vi "Configure Channels.vi"(8 "error in":errorcluster, 11 "DIO DAQmx PWM CFG in":refnum<class "CO DAQmx PWM CFG.lvclass">) -> (0 "error out":errorcluster, 3 "DIO DAQmx PWM CFG out":refnum<class "CO DAQmx PWM CFG.lvclass">)   [LabVIEW 2023, in "CO DAQmx PWM CFG.lvclass"]
uses:
  CO DAQmx PWM CFG.lvclass
  CO DAQmx PWM CFG.lvclass/CO DAQmx PWM CFG.ctl
  <vilib>/Utility/error.llb/Error Cluster From Error Code.vi
  <vilib>/ErrorRing/Error Ring.xnode
  Configuration/Configuration JSON/Configuration JSON Base/CFG JSON.lvclass
  DAQmx/DAQmx Base CFG/DAQmx Base CFG.lvclass
  <vilib>/DAQmx/create/channels.llb/DAQmx Create Channel (CO-Pulse Generation-Frequency).vi
  9b4e2dbf-c434-4eef-b69c-50b2f8d92478.vi
panel:
  out "Idle State":i32(ring)=10214 items=["High"=10192, "Low"=10214]
  out "Units":i32(ring)=10373 items=["Hz"=10373]
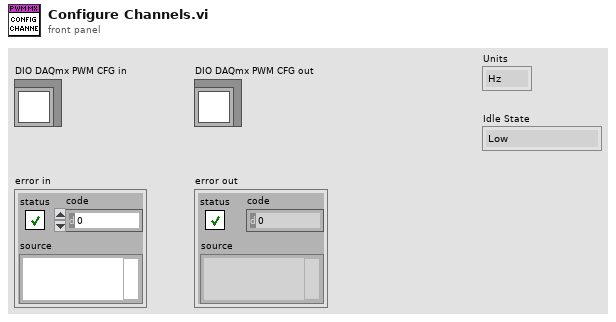
[diagram p1: front panel]
types:
  T1 = cluster{"Name":string, "Enabled":bool, "Duty Cycle":dbl, "Frequency":dbl, "Units":string, "Idle State":string, "Initial Delay":dbl}[]
  T2 = typedef "LVStringsAndValuesArrayTypeDef_I32.ctl" = cluster{"String":string, "Value":i32}[]
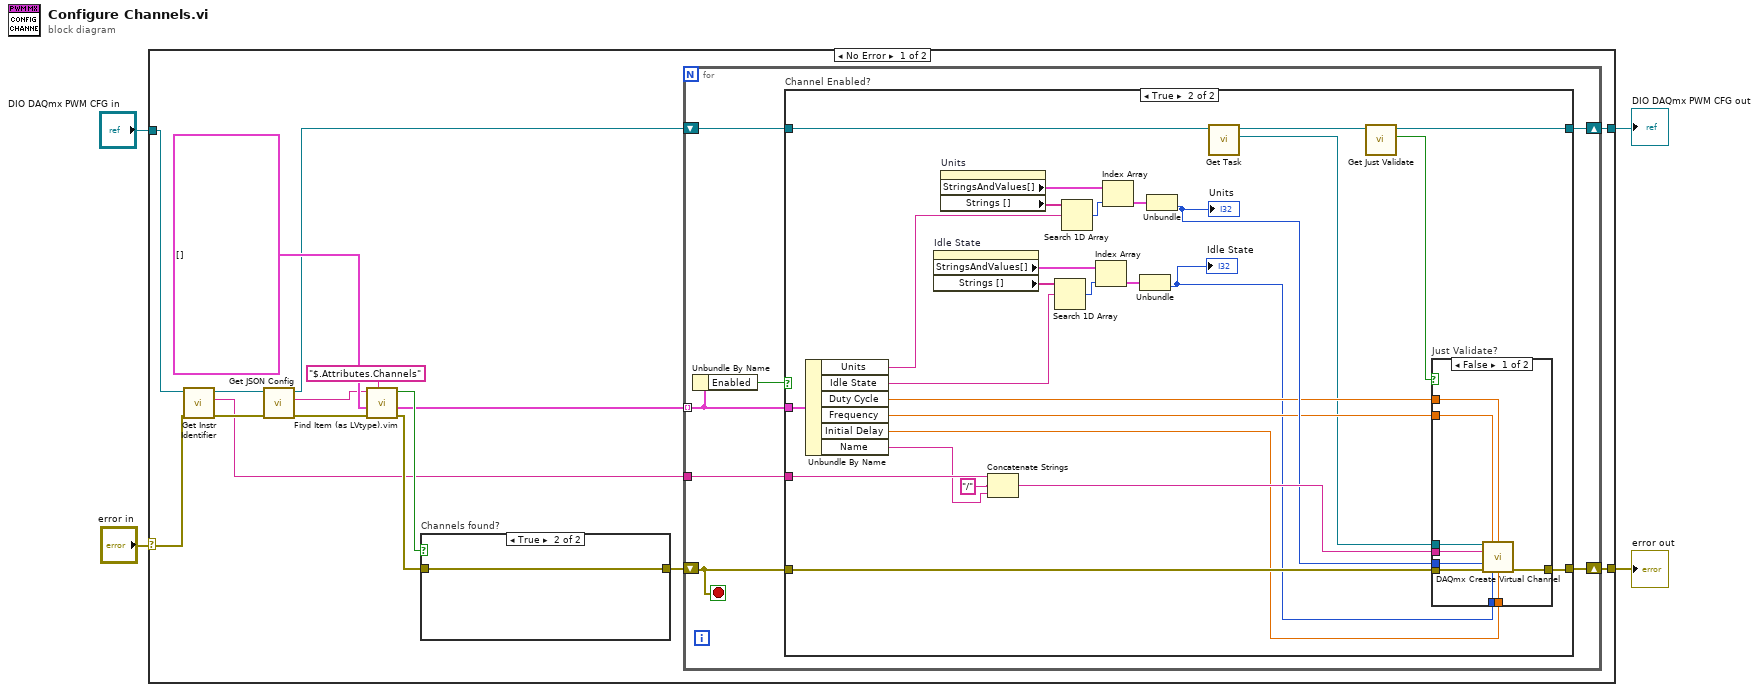
[diagram p0: block diagram]
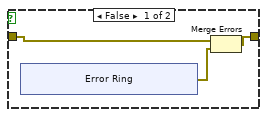
[diagram p4: hidden frame]
diagram:
  n1 = case shown="No Error" "error in" {
    selector: "error in" -> [w5 w76]
    tunnel: "DIO DAQmx PWM CFG in" -> [w9 w77]
    tunnel: [w8 w76] -> w3
    tunnel: [w6 w77] -> w2
    frame No Error {
      n2 = call-dynamic "Get Instr Identifier.vi"("error in (no error)"=w5, "Configuration Base in"=w9) -> ("error out"=w12:errorcluster, "Instr Ident"=w10:string, "Configuration Base out"=w11:refnum<class "CO DAQmx PWM CFG.lvclass">)  [unwired: 7 in]
      n3 = call "Get JSON Config.vi"("error in (no error)"=w12, "CFG Base in"=w11) -> ("error out"=w19:errorcluster, "<JSON>Config>"=w13:string, "CFG Base out"=w7:refnum<class "CO DAQmx PWM CFG.lvclass">)  [unwired: 7 in]
      n4 = call "Find Item (as LVtype).vim"("$Path or Item Name"="$.Attributes.Channels", "error in (no error)"=w19, "Data Type and Default Value"=T1 [], "JSON"=w13) -> ("error out"=w17:errorcluster, "Data"=w15:T1, "Found"=w18:bool)  [unwired: 4 in, 1 out]
      n5 = case "Channels found?" shown="True" w18 {
        tunnel: w17 -> [w69 w75]
        tunnel: [w67 w75] -> w16
        frame False {
          n6 = xnode "Error Ring"() -> ("error out"=w68:errorcluster)
          n7 = Merge Errors(w69, w68) -> (w67:errorcluster)
        }
        frame True {
        }
      }
      n8 = for {
        tunnel: w15 -> [w24] mode=indexing
        shift-right: [w27] -> w8
        shift-left: w16 -> [w26]
        tunnel: w10 -> [w25]
        shift-right: [w22] -> w6
        shift-left: w7 -> [w21]
        stop <- w26 stop-if-true
        n9 = Unbundle By Name(w24) -> ("Enabled"=w23:bool)
        n10 = case "Channel Enabled?" shown="True" w23 {
          tunnel: [w29 w34] -> w27
          tunnel: w26 -> [w29 w49]
          tunnel: w25 -> [_ w47]
          tunnel: w24 -> [_ w45]
          tunnel: [w28 w31] -> w22
          tunnel: w21 -> [w28 w32]
          frame False {
          }
          frame True {
            n11 = Unbundle By Name(w45) -> ("Units"=w50:string, "Idle State"=w40:string, "Duty Cycle"=w39:dbl, "Frequency"=w38:dbl, "Initial Delay"=w36:dbl, "Name"=w46:string)
            n12 = property on="Idle State" class="Ring (strict)"() -> ("StringsAndValues[]"=w56:T2, "Strings []"=w42:string[])  [unwired: 2 in, 2 out]
            n13 = property on="Units" class="Ring (strict)"() -> ("StringsAndValues[]"=w52:T2, "Strings []"=w51:string[])  [unwired: 2 in, 2 out]
            n14 = Concatenate Strings(w47, "/" ("string"), w46) -> (w44:string)
            n15 = Search 1D Array(1D array=w42, element=w40) -> (index of element=w41:i32)  [unwired: 1 in]
            n16 = Search 1D Array(1D array=w51, element=w50) -> (index of element=w53:i32)  [unwired: 1 in]
            n17 = Index Array(array=w56, index=w41) -> (element=w55:cluster{"String":string, "Value":i32})
            n18 = Index Array(array=w52, index=w53) -> (element=w54:cluster{"String":string, "Value":i32})
            n19 = Unbundle(w55) -> ("Value"=w37:i32)  [unwired: 1 out]
            "Idle State" <- w37
            n20 = Unbundle(w54) -> ("Value"=w43:i32)  [unwired: 1 out]
            "Units" <- w43
            n21 = call "Get Task.vi"("DAQmx Base CFG in"=w32) -> ("Task"=w35:refnum<k21>, "DAQmx Base CFG out"=w33:refnum<class "CO DAQmx PWM CFG.lvclass">)  [unwired: 8 in, 1 out]
            n22 = call "Get Just Validate.vi"("CFG JSON Base in"=w33) -> ("Just Validate"=w30:bool, "CFG JSON Base out"=w31:refnum<class "CO DAQmx PWM CFG.lvclass">)  [unwired: 8 in, 1 out]
            n23 = case "Just Validate?" shown="False" w30 {
              tunnel: w49 -> [w65 w66]
              tunnel: w44 -> [w64 _]
              tunnel: w43 -> [w63 _]
              tunnel: w39 -> [w62 _]
              tunnel: w38 -> [w61 _]
              tunnel: w37 -> [w60 _]
              tunnel: w36 -> [w59 _]
              tunnel: w35 -> [w58 _]
              tunnel: [w57 w66] -> w34
              frame False {
                n24 = call-poly <vilib>:"DAQmx Create Virtual Channel.vi"("task in"=w58, "frequency"=w61, "duty cycle"=w62, "counter"=w64, "units"=w63, "error in"=w65, "idle state"=w60, "initial delay"=w59) -> ("error out"=w57:errorcluster)  [unwired: 6 in, 1 out]
              }
              frame True {
              }
            }
          }
        }
      }
    }
    frame Error {
    }
  }
  "error out" <- w3
  "DIO DAQmx PWM CFG out" <- w2
